vi "Write to TDMS.vi"(8 "error in (no error)":errorcluster, 10 "TDMS File Ref":refnum<k34>, 11 "2D String Logging Data in":refnum<class "2D String Logging Data.lvclass">) -> (0 "error out":errorcluster)   [LabVIEW 2024, in "Logging Data.lvlib" / "2D String Logging Data.lvclass"]
uses:
  2D String Logging Data.lvclass
  2D String Logging Data.lvclass/2D String Logging Data.ctl
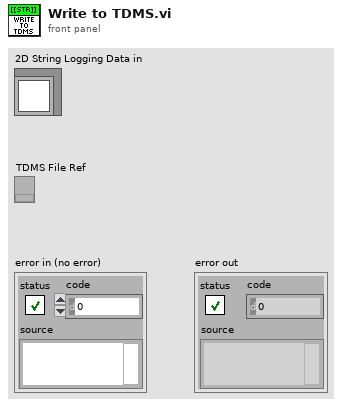
[diagram p1: front panel]
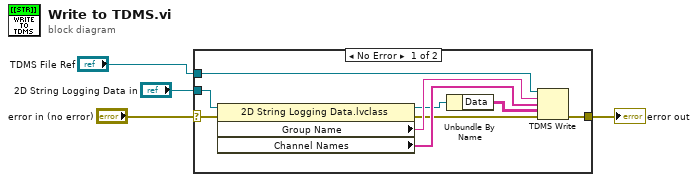
[diagram p0: block diagram]
diagram:
  n1 = case shown="No Error" "error in (no error)" {
    selector: "error in (no error)" -> [w6 w14]
    tunnel: "2D String Logging Data in" -> [w13 _]
    tunnel: "TDMS File Ref" -> [w7 _]
    tunnel: [w5 w14] -> w1
    frame No Error {
      n2 = property class="2D String Logging Data.lvclass"(reference=w13, error in=w6) -> (reference out=w9:refnum<class "2D String Logging Data.lvclass">, error out=w10:errorcluster, "Group Name"=w12:string, "Channel Names"=w11:string[])
      n3 = Unbundle By Name(w9) -> ("Data"=w8:string[][])
      n4 = TDMS Write(0:w7, 5:w12, 7:w11, 9:w8, 11:w10) -> (15:w5:errorcluster)  [unwired: 1 in, 3 out]
    }
    frame Error {
    }
  }
  "error out" <- w1
